vi "Get SpreadsheetDocument Refnum.vi"(8 "error in (no error)":errorcluster, 11 "ooCalc in":refnum<class "ooCalc.lvclass">) -> (0 "error out":errorcluster, 1 "SpreadsheetDocument":refnum<k24>, 3 "ooCalc out":refnum<class "ooCalc.lvclass">)   [LabVIEW 2009, in "ooCalc.lvclass"]
uses:
  ooCalc.lvclass
  C:/Projets/LAVAG/OpenOfficeRGT/AODL/DLLs/AODL.dll
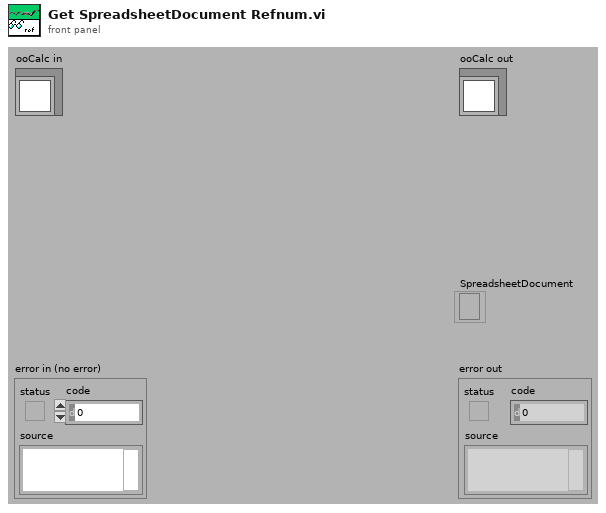
[diagram p1: front panel]
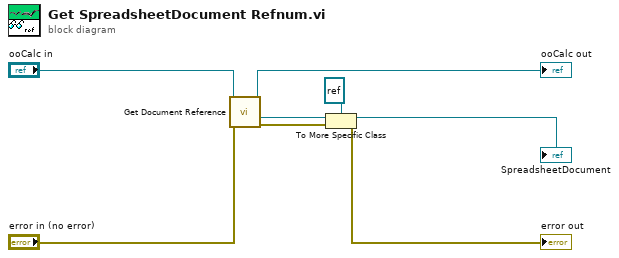
[diagram p0: block diagram]
diagram:
  n1 = call-dynamic "Get Document Reference.vi"("error in (no error)"="error in (no error)", "ooDocument in"="ooCalc in") -> ("error out"=w6:errorcluster, "Document"=w7:refnum<k24>, "ooDocument out"=→"ooCalc out":refnum<class "ooCalc.lvclass">)  [unwired: 7 in]
  n2 = To More Specific Class(target class=refnum<k24> refnum ("ooCalc.Document"), reference=w7, error in=w6) -> (specific class reference=→"SpreadsheetDocument":refnum<k24>, error out=→"error out":errorcluster)
